vi "Interpolation (Control - Window Init Mem - Wave Init Mem - Graph) Test.vi"() -> ()   [LabVIEW 2014]
uses:
  <vilib>/rvi/interface/nirviOpenFPGA/nirviOpenFPGA.xnode
  <vilib>/rvi/interface/nirviMethod/nirviMethod.xnode
  <vilib>/FPGAPlugInAG/Dynamic/niLvFpga_ConfigureFifo_Dynamic.vi
  <vilib>/rvi/errors/niLvFpgaMergeErrorWithErrorCode.vi
  <vilib>/FPGAPlugInAG/Dynamic/niLvFpga_StartFifo_Dynamic.vi
  <vilib>/FPGAPlugInAG/Dynamic/niLvFpga_Run_Dynamic.vi
  <vilib>/FPGAPlugInAG/Dynamic/niLvFpga_Abort_Dynamic.vi
  <vilib>/rvi/interface/nirviCloseFPGA/nirviCloseFPGA.xnode
  <vilib>/rvi/interface/nirviReadWriteControl/nirviReadWriteControl.xnode
  <vilib>/rvi/interface/Simulation/niFpgaSimulationCallBeginRW.vi
  <vilib>/rvi/errors/niLvFpgaAdjustHostInterfaceError.vi
  NiFpgaLv.dll
  <vilib>/Utility/error.llb/Error Cluster From Error Code.vi
  <vilib>/FPGAPlugInAG/Dynamic/niLvFpga_ReadFifo_Dynamic.vi
  <vilib>/FPGAPlugInAG/Dynamic/niLvFpga_Close_Dynamic.vi
  FPGA Bitfiles/LaserDistanceSen_FPGATarget_DoubleFFTMesuram_j5IMksq1wkg.lvbitx
  FPGA Target/Test VIs/Double FFT Mesurament (Max Bin detection - Control - Windowing - Init Wave - Graph) test.vi
  <vilib>/FPGAPlugInAG/sbRIO-9636/niLvFpga_Open_sbRIO-9636.vi
  <vilib>/rvi/interface/common/dynamic/niFpgaDynamicAddResources.vi
panel:
  out "FFT (freq)":waveform(dbl)(graph)
  out "Signal (points)":dbl[](graph)
  out "Signal (t)":waveform(dbl)(graph)
  out "FFT (bin)":dbl[](graph)
  in  "Snapshot":bool
  out "Ftone+":dbl
  out "Ftone-":dbl
  in  "Windowing":T1(ring)
  in  "first bin":i32=10
  in  "last bin":i32=255
  in  "lower limit 2":u32(slide)=677 scale=625.0..737.0
  in  "lower limit 1":u32(slide)=59 scale=0.0..112.0
  out "Detected Frequency Tone - (Hz)":dbl
  in  "stop":bool
  out "Max Bin":i32
  out "Max Amp":dbl format="%.2f"
  out "Prev Bin":i32
  out "Next Bin":i32
  out "Prev Amp":dbl format="%.2f"
  out "Next Amp":dbl format="%.2f"
  out "Interpolated Bin":dbl
  in  "Interpolation Method":T2(ring)=enum."Jain"
  # "WARNING:\nOnce pressed wait untill the end of operation"
  # "ONLINE parameter"
  # "OFFLINE parameters"
  # "Max Detection FFT bin range"
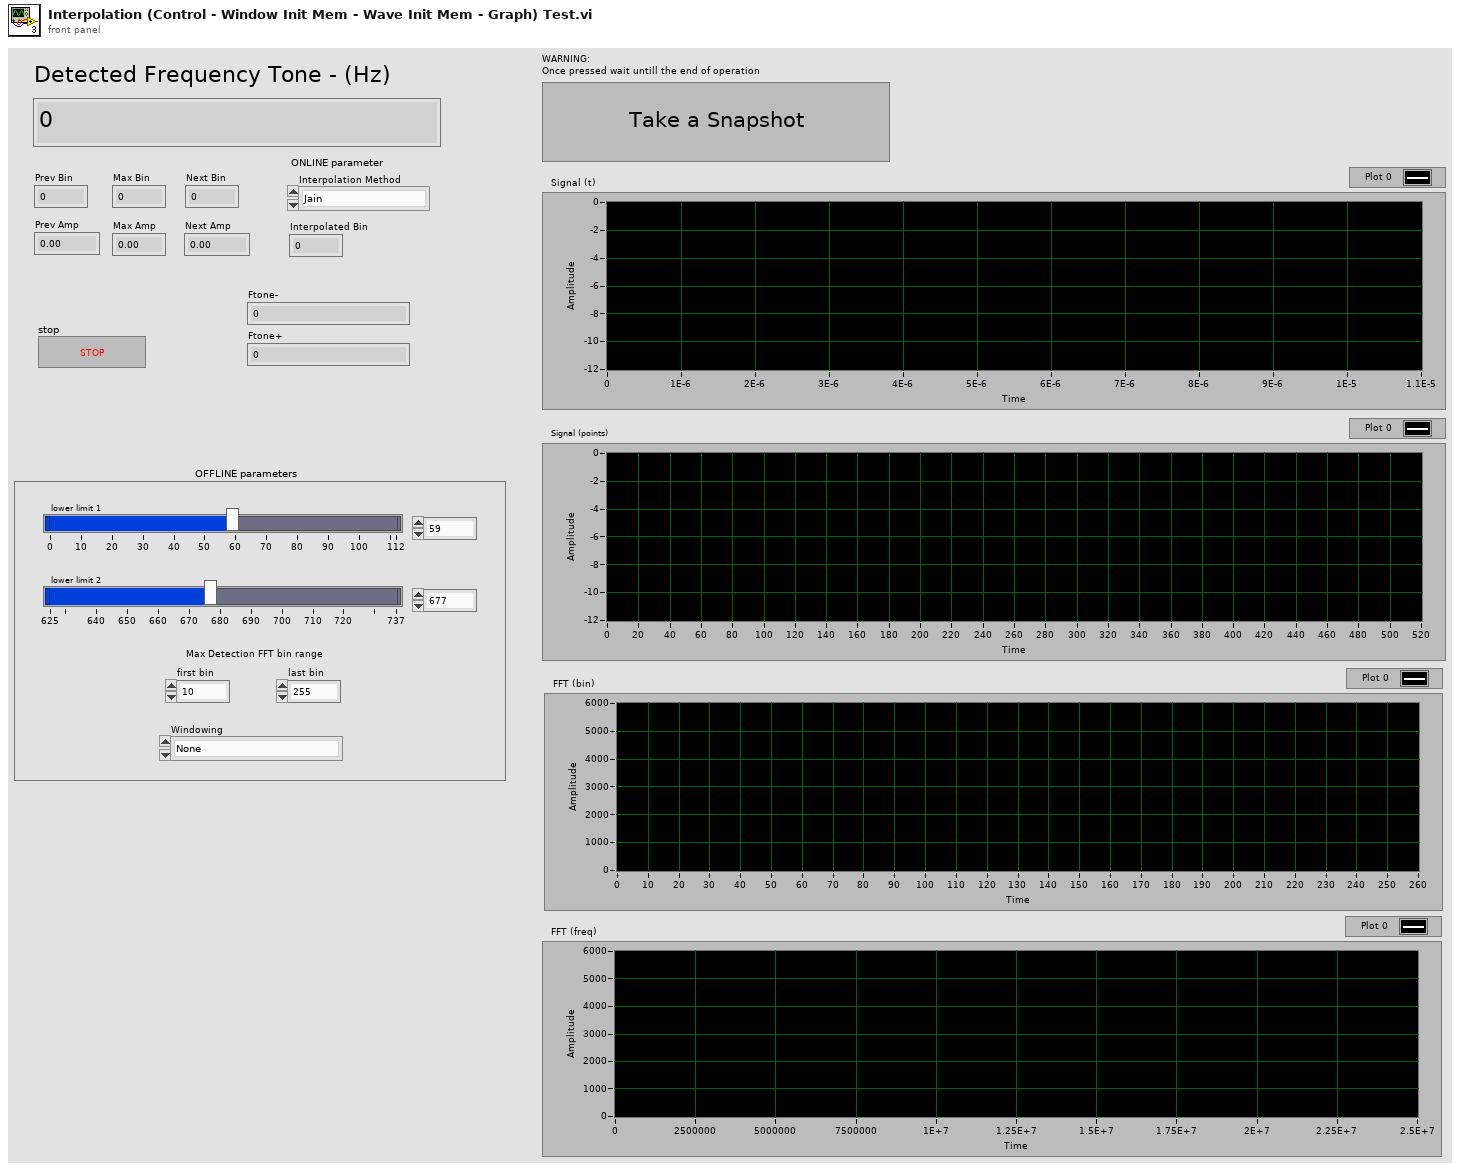
[diagram p1: front panel]
types:
  T1 = enum16{"None", "Hanning", "Hamming", "Blackman", "Blackman-Harris"}
  T2 = enum16{"Quadratic", "McLeodd", "Barycentric", "Jain"}
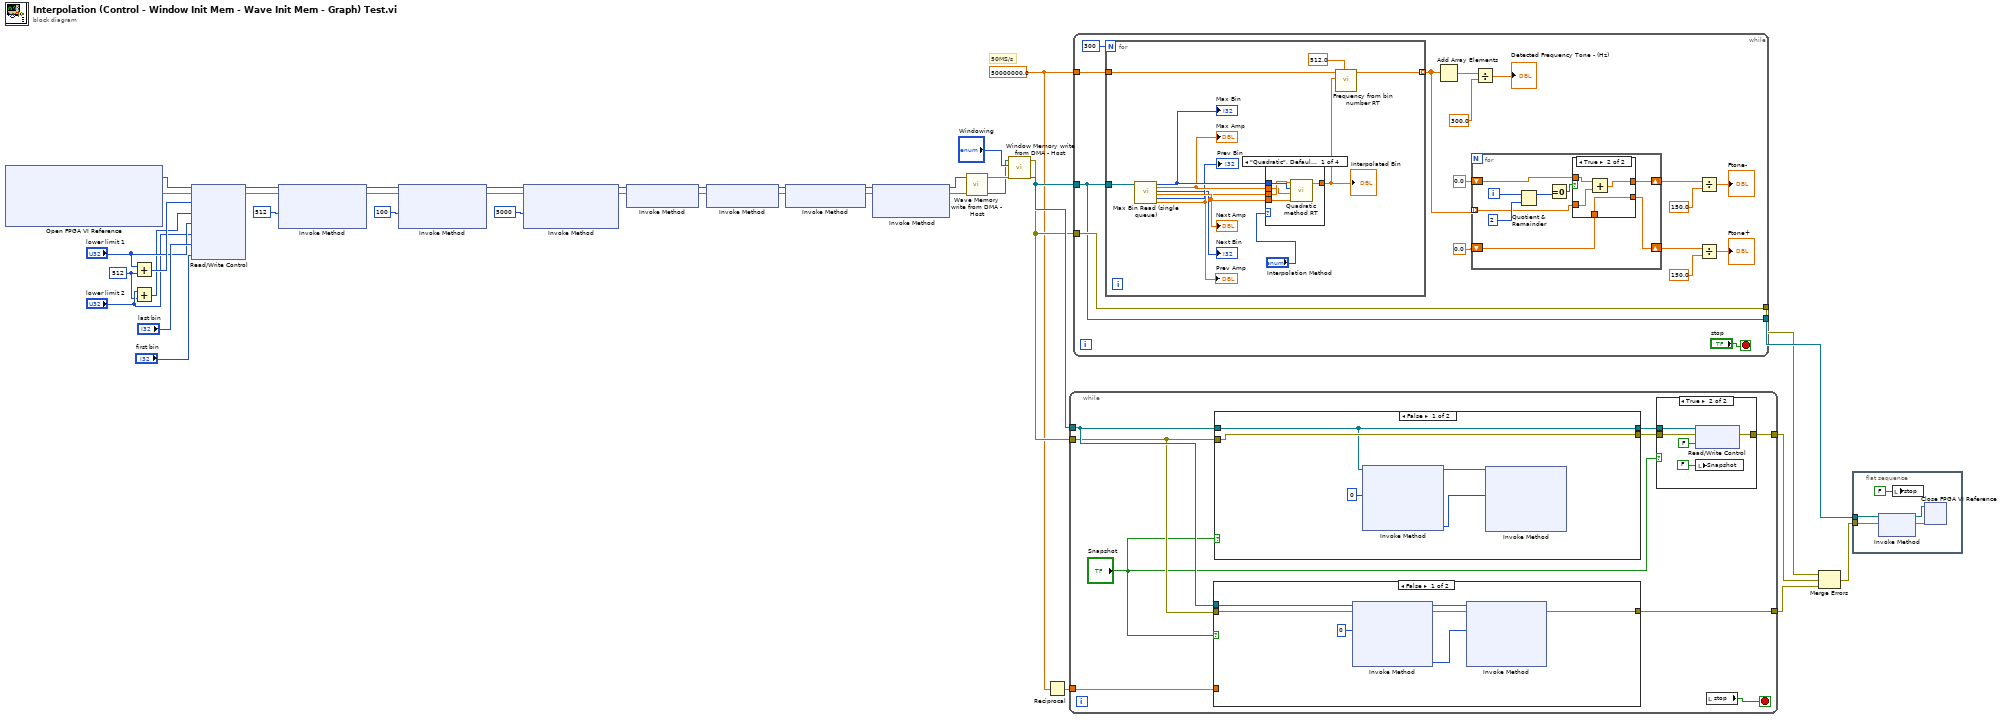
[diagram p0: block diagram]
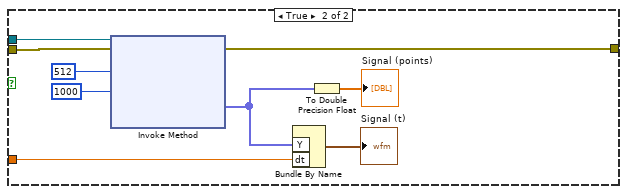
[diagram p3: hidden frame]
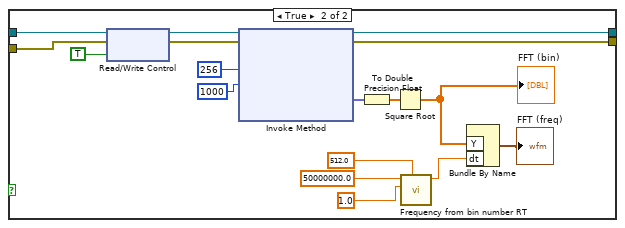
[diagram p4: hidden frame]
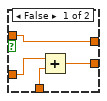
[diagram p5: hidden frame]
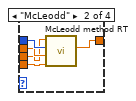
[diagram p6: hidden frame]
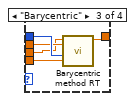
[diagram p7: hidden frame]
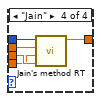
[diagram p8: hidden frame]
diagram:
  w34 = u32 512 ("y")
  w9 = 50000000.0 ("Sample Rate (S/s)")
  # "50MS/s"
  n1 = xnode "Open FPGA VI Reference"() -> ("FPGA VI Reference Out"=w33:refnum<k20>, "error out"=w32:errorcluster)  [unwired: 2 in]
  n2 = Add(x="lower limit 1", y=w34) -> (x+y=w38:u32)
  n3 = Add(x="lower limit 2", y=w34) -> (x+y=w36:u32)
  n4 = xnode "Read/Write Control"("FPGA VI Reference In"=w33, "error in"=w32, "upper limit 1"=w38, "upper limit 2"=w36, "lower limit 1"="lower limit 1", "lower limit 2"="lower limit 2", "last bin"="last bin", "first bin"="first bin") -> ("FPGA VI Reference Out"=w27:refnum<k20>, "error out"=w26:errorcluster)
  n5 = xnode "Invoke Method"("FPGA VI Reference In"=w27, "error in"=w26, "Requested Depth"=u32 512) -> ("FPGA VI Reference Out"=w25:refnum<k20>, "error out"=w24:errorcluster)  [unwired: 1 out]
  n6 = xnode "Invoke Method"("FPGA VI Reference In"=w25, "error in"=w24, "Requested Depth"=u32 100) -> ("FPGA VI Reference Out"=w23:refnum<k20>, "error out"=w22:errorcluster)  [unwired: 1 out]
  n7 = xnode "Invoke Method"("FPGA VI Reference In"=w23, "error in"=w22, "Requested Depth"=u32 5000) -> ("FPGA VI Reference Out"=w3:refnum<k20>, "error out"=w4:errorcluster)  [unwired: 1 out]
  n8 = xnode "Invoke Method"("FPGA VI Reference In"=w3, "error in"=w4) -> ("FPGA VI Reference Out"=w16:refnum<k20>, "error out"=w15:errorcluster)
  n9 = xnode "Invoke Method"("FPGA VI Reference In"=w16, "error in"=w15) -> ("FPGA VI Reference Out"=w18:refnum<k20>, "error out"=w17:errorcluster)
  n10 = xnode "Invoke Method"("FPGA VI Reference In"=w18, "error in"=w17) -> ("FPGA VI Reference Out"=w1:refnum<k20>, "error out"=w2:errorcluster)
  n11 = xnode "Invoke Method"("FPGA VI Reference In"=w1, "error in"=w2) -> ("FPGA VI Reference Out"=w8:refnum<k20>, "error out"=w7:errorcluster)  [unwired: 1 in]
  n12 = call "Wave Memory write from DMA - Host.vi"("error in"=w7, "FPGA VI Reference In"=w8) -> ("FPGA VI Reference Out"=w5:refnum<k20>, "error out"=w6:errorcluster)  [unwired: 7 in, 1 out]
  n13 = call "Window Memory write from DMA - Host.vi"("error in"=w6, "Enum"="Windowing", "FPGA VI Reference In"=w5) -> ("FPGA VI Reference Out"=w29:refnum<k20>, "error out"=w28:errorcluster)  [unwired: 5 in, 2 out]
  n14 = Reciprocal(x=w9) -> (1/x=w10:dbl)
  n15 = while {
    tunnel: w29 -> [w49]
    tunnel: w28 -> [w48]
    tunnel: [w45] -> w14
    tunnel: [w44] -> w13
    tunnel: w10 -> [w42]
    stop <- w47 stop-if-true
    n16 = case shown="False" "Snapshot" {
      tunnel: w49 -> [w61 w71]
      tunnel: w48 -> [w59 w70]
      tunnel: [w58 w67] -> w44
      tunnel: w42 -> [_ w65]
      frame False {
        n17 = xnode "Invoke Method"("FPGA VI Reference In"=w61, "error in"=w59, "Number of Elements"=u32 0) -> ("FPGA VI Reference Out"=w57:refnum<k20>, "error out"=w56:errorcluster, "Elements Remaining"=w60:u32)  [unwired: 1 in, 1 out]
        n18 = xnode "Invoke Method"("FPGA VI Reference In"=w57, "error in"=w56, "Number of Elements"=w60) -> ("error out"=w58:errorcluster)  [unwired: 1 in, 3 out]
      }
      frame True {
        n19 = xnode "Invoke Method"("FPGA VI Reference In"=w71, "error in"=w70, "Number of Elements"=u32 512, "Timeout (ms)"=1000) -> ("error out"=w67:errorcluster, "Data"=w64:fxp<+/-,12,12>[])  [unwired: 2 out]
        n20 = Bundle By Name("Y"=w64, "dt"=w65) -> (→"Signal (t)":waveform(dbl))  [unwired: 1 in]
        n21 = To Double Precision Float(number=w64) -> (double precision float=→"Signal (points)":dbl[])
      }
    }
    n22 = case shown="False" "Snapshot" {
      tunnel: w49 -> [w74 w93]
      tunnel: w48 -> [w76 w92]
      tunnel: [w76 w91] -> w46
      tunnel: [w74 w90] -> w43
      frame False {
        n23 = xnode "Invoke Method"("FPGA VI Reference In"=w74, "Number of Elements"=u32 0) -> ("FPGA VI Reference Out"=w72:refnum<k20>, "Elements Remaining"=w73:u32)  [unwired: 2 in, 2 out]
        n24 = xnode "Invoke Method"("FPGA VI Reference In"=w72, "Number of Elements"=w73) -> ()  [unwired: 2 in, 4 out]
      }
      frame True {
        n25 = xnode "Read/Write Control"("FPGA VI Reference In"=w93, "error in"=w92, "snapshot"=TRUE) -> ("FPGA VI Reference Out"=w88:refnum<k20>, "error out"=w87:errorcluster)
        n26 = xnode "Invoke Method"("FPGA VI Reference In"=w88, "error in"=w87, "Number of Elements"=u32 256, "Timeout (ms)"=1000) -> ("FPGA VI Reference Out"=w90:refnum<k20>, "error out"=w91:errorcluster, "Data"=w84:fxp<+,44,44>[])  [unwired: 1 out]
        n27 = To Double Precision Float(number=w84) -> (double precision float=w83:dbl[])
        n28 = Square Root(x=w83) -> (sqrt(x)=w78:dbl[])
        "FFT (bin)" <- w78
        n29 = call "Frequency from bin number RT.vi"("FFT size"=512.0, "Bin number"=1.0, "Sample Rate (S/s)"=50000000.0) -> ("Detected Frequency (Hz)"=w79:dbl)  [unwired: 8 in]
        n30 = Bundle By Name("Y"=w78, "dt"=w79) -> (→"FFT (freq)":waveform(dbl))  [unwired: 1 in]
      }
    }
    n31 = case shown="True" "Snapshot" {
      tunnel: w46 -> [w50 w55]
      tunnel: [w50 w54] -> w45
      tunnel: w43 -> [_ w53]
      frame False {
      }
      frame True {
        n32 = xnode "Read/Write Control"("FPGA VI Reference In"=w53, "error in"=w55, "snapshot"=FALSE) -> ("error out"=w54:errorcluster)  [unwired: 1 out]
        n33 = local write "Snapshot"(FALSE ("Snapshot")) -> ()
      }
    }
    n34 = local read "stop"() -> (w47:bool)
  }
  n35 = while {
    tunnel: w9 -> [w109]
    tunnel: w29 -> [w94]
    tunnel: w28 -> [w95]
    tunnel: [w94] -> w31
    tunnel: [w95] -> w12
    stop <- "stop" stop-if-true
    n36 = for {
      N: 300 -> [_]
      tunnel: w94 -> [w134]
      tunnel: w109 -> [w137]
      tunnel: [w135] -> w101 mode=indexing
      n37 = call "Max Bin Read (single queue).vi"("FPGA VI Reference In"=w134) -> ("Max Bin"=w133:i32, "Max Amp"=w132:dbl, "Next Bin"=→"Next Bin":i32, "Next Amp"=w131:dbl, "Prev Bin"=→"Prev Bin":i32, "Prev Amp"=w130:dbl)  [unwired: 13 in]
      "Max Bin" <- w133
      "Max Amp" <- w132
      "Prev Amp" <- w130
      "Next Amp" <- w131
      n38 = case shown="\"Quadratic\", Default" "Interpolation Method" {
        tunnel: w133 -> [w143 w148 w153 w158]
        tunnel: w132 -> [w140 w147 w152 w157]
        tunnel: w130 -> [w141 w146 w151 w156]
        tunnel: w131 -> [w142 w145 w150 w155]
        tunnel: [w144 w149 w154 w159] -> w136
        frame "Quadratic", Default {
          n39 = call "Quadratic method RT.vi"("Next Amplitude"=w142, "Max Amplitude"=w140, "Max bin"=w143, "Prev Amplitude"=w141) -> ("Bin"=w144:dbl)  [unwired: 7 in]
        }
        frame "McLeodd" {
          n40 = call "McLeodd method RT.vi"("Next Amp"=w145, "Max Amp"=w147, "Max Bin"=w148, "Prev Amp"=w146) -> ("Bin"=w149:dbl)  [unwired: 7 in]
        }
        frame "Barycentric" {
          n41 = call "Barycentric method RT.vi"("Next Amp"=w150, "Max Bin"=w153, "Max Amp"=w152, "Prev Amp"=w151) -> ("Bin"=w154:dbl)  [unwired: 7 in]
        }
        frame "Jain" {
          n42 = call "Jain's method RT.vi"("Prev Amp"=w156, "Next Amp"=w155, "Max Amp"=w157, "Max Bin"=w158) -> ("Bin"=w159:dbl)  [unwired: 7 in]
        }
      }
      "Interpolated Bin" <- w136
      n43 = call "Frequency from bin number RT.vi"("FFT size"=512.0, "Bin number"=w136, "Sample Rate (S/s)"=w137) -> ("Detected Frequency (Hz)"=w135:dbl)  [unwired: 8 in]
    }
    n44 = Add Array Elements(numeric array=w101) -> (sum=w108:dbl)
    n45 = for {
      tunnel: w101 -> [w114] mode=indexing
      shift-right: [w113] -> w104
      shift-left: 0.0 -> [w115]
      shift-right: [w111] -> w97
      shift-left: 0.0 -> [w112]
      i -> [w119]
      n46 = Quotient & Remainder(x=w119, y=2) -> (x-y*floor(x/y)=w117:i32)  [unwired: 1 out]
      n47 = Equal To 0?(x=w117) -> (x = 0?=w116:bool)
      n48 = case shown="True" w116 {
        tunnel: w115 -> [w123 w127]
        tunnel: w114 -> [w122 w126]
        tunnel: [w123 w125] -> w113
        tunnel: w112 -> [w121 w124]
        tunnel: [w120 w124] -> w111
        frame False {
          n49 = Add(x=w122, y=w121) -> (x+y=w120:dbl)
        }
        frame True {
          n50 = Add(x=w127, y=w126) -> (x+y=w125:dbl)
        }
      }
    }
    n51 = Divide(x=w108, y=300.0) -> (x/y=→"Detected Frequency Tone - (Hz)":dbl)
    n52 = Divide(x=w104, y=150.0) -> (x/y=→"Ftone-":dbl)
    n53 = Divide(x=w97, y=150.0) -> (x/y=→"Ftone+":dbl)
  }
  n54 = Merge Errors(w12, w14, w13) -> (w11:errorcluster)
  n55 = flat-sequence {
    tunnel: w31 -> [w162]
    tunnel: w11 -> [w161]
    frame #0 {
      n56 = xnode "Invoke Method"("FPGA VI Reference In"=w162, "error in"=w161) -> ("FPGA VI Reference Out"=w163:refnum<k20>, "error out"=w164:errorcluster)
      n57 = local write "stop"(FALSE ("stop")) -> ()
      n58 = xnode "Close FPGA VI Reference"("FPGA VI Reference In"=w163, "error in"=w164) -> ()  [unwired: 1 out]
    }
  }
